vi "Frontpanel.vi"() -> ()   [LabVIEW 2015]
panel:
  in  "stop":bool
  in  "Zeile":u32
  in  "xyz":dbl[](array[numeric])
  in  "Lšschen":bool
  in  "Laden":bool
  in  "Speichern":bool
  in  "Bemerkung":string
  in  "Wellenl.":string
  in  "Favoriten":i32(listbox)
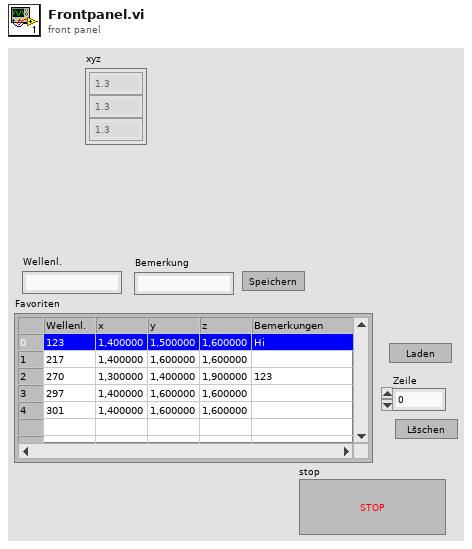
[diagram p1: front panel]
types:
  T1 = enum16{"None", "On Hover", "On Key Focus", "On Hover or Key Focus"}
  T2 = cluster{string[][], "element":string[], string[]}
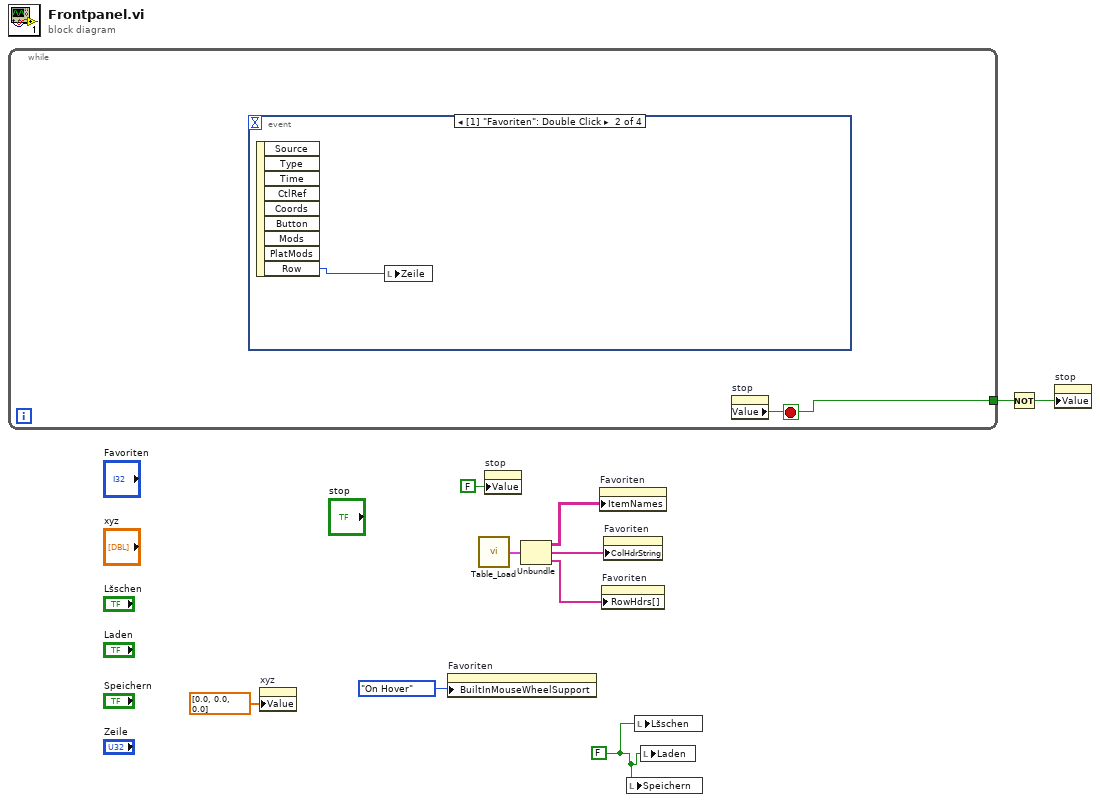
[diagram p0: block diagram]
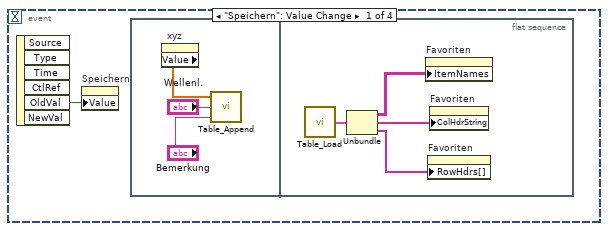
[diagram p2: hidden frame]
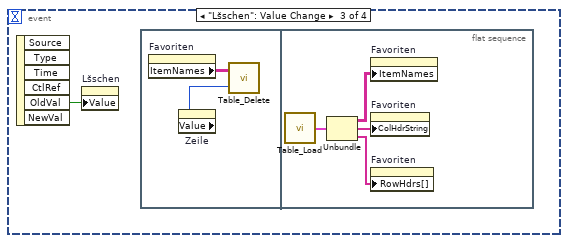
[diagram p3: hidden frame]
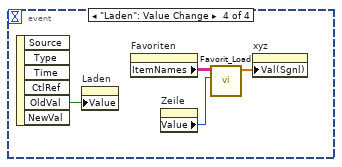
[diagram p4: hidden frame]
diagram:
  w2 = FALSE ("Speichern")
  n1 = while {
    tunnel: [w11] -> w10
    stop <- w11 stop-if-true
    n2 = event shown="[1] \"Favoriten\": Double Click" {
      selector: _ -> [_ _ _ _]
      dyn-events: _ -> [_ _ _ _]
      timeout: _ -> [_ _ _ _]
      event "Speichern": Value Change {
        n3 = event-data() -> ("OldVal"=w12:bool)  [unwired: 1 in, 5 out]
        n4 = property on="Speichern" class="Bool (strict)"("Value"=w12) -> ()  [unwired: 2 in, 2 out]
        n5 = flat-sequence {
          frame #0 {
            n6 = property on="xyz" class="Arr (strict)"() -> ("Value"=w15:dbl[])  [unwired: 2 in, 2 out]
            n7 = call "Table_Append.vi"("Bemerkung"="Bemerkung", "WellenlŠnge"="Wellenl.", "initialized array"=w15) -> ()  [unwired: 1 in]
          }
          frame #1 {
            n8 = call "Table_Load.vi"() -> ("output cluster"=w19:T2)  [unwired: 1 in]
            n9 = Unbundle(w19) -> (w18:string[][], "element"=w16:string[], w17:string[])
            n10 = property on="Favoriten" class="MCListbox (strict)"("ItemNames"=w18) -> ()  [unwired: 2 in, 2 out]
            n11 = property on="Favoriten" class="MCListbox (strict)"("RowHdrs[]"=w17) -> ()  [unwired: 2 in, 2 out]
            n12 = property on="Favoriten" class="MCListbox (strict)"("ColHdrString"=w16) -> ()  [unwired: 2 in, 2 out]
          }
        }
      }
      event "Favoriten": Double Click {
        n13 = event-data() -> ("Row"=w20:i32)  [unwired: 1 in, 8 out]
        n14 = local write "Zeile"(w20) -> ()
      }
      event "Lšschen": Value Change {
        n15 = event-data() -> ("OldVal"=w21:bool)  [unwired: 1 in, 5 out]
        n16 = property on="Lšschen" class="Bool (strict)"("Value"=w21) -> ()  [unwired: 2 in, 2 out]
        n17 = flat-sequence {
          frame #0 {
            n18 = property on="Favoriten" class="MCListbox (strict)"() -> ("ItemNames"=w23:string[][])  [unwired: 2 in, 2 out]
            n19 = property on="Zeile" class="DigNum (strict)"() -> ("Value"=w22:u32)  [unwired: 2 in, 2 out]
            n20 = call "Table_Delete.vi"("Zeile"=w22, "Item Names"=w23) -> ()  [unwired: 1 in]
          }
          frame #1 {
            n21 = call "Table_Load.vi"() -> ("output cluster"=w27:T2)  [unwired: 1 in]
            n22 = Unbundle(w27) -> (w26:string[][], "element"=w24:string[], w25:string[])
            n23 = property on="Favoriten" class="MCListbox (strict)"("ItemNames"=w26) -> ()  [unwired: 2 in, 2 out]
            n24 = property on="Favoriten" class="MCListbox (strict)"("ColHdrString"=w24) -> ()  [unwired: 2 in, 2 out]
            n25 = property on="Favoriten" class="MCListbox (strict)"("RowHdrs[]"=w25) -> ()  [unwired: 2 in, 2 out]
          }
        }
      }
      event "Laden": Value Change {
        n26 = event-data() -> ("OldVal"=w31:bool)  [unwired: 1 in, 5 out]
        n27 = property on="Laden" class="Bool (strict)"("Value"=w31) -> ()  [unwired: 2 in, 2 out]
        n28 = property on="Favoriten" class="MCListbox (strict)"() -> ("ItemNames"=w29:string[][])  [unwired: 2 in, 2 out]
        n29 = property on="Zeile" class="DigNum (strict)"() -> ("Value"=w30:u32)  [unwired: 2 in, 2 out]
        n30 = call "Favorit_Load.vi"("Value"=w30, "ItemNames"=w29) -> ("Array"=w28:dbl[])  [unwired: 9 in]
        n31 = property on="xyz" class="Arr (strict)"("Val(Sgnl)"=w28) -> ()  [unwired: 2 in, 2 out]
      }
    }
    n32 = property on="stop" class="Bool (strict)"() -> ("Value"=w11:bool)  [unwired: 2 in, 2 out]
  }
  n33 = property on="xyz" class="Arr (strict)"("Value"=dbl[] [0.0, 0.0, 0.0] ("Array")) -> ()  [unwired: 2 in, 2 out]
  n34 = property on="Favoriten" class="MCListbox (strict)"("BuiltInMouseWheelSupport"=T1."On Hover" ("Built-In Mouse Wheel Support")) -> ()  [unwired: 2 in, 2 out]
  n35 = call "Table_Load.vi"() -> ("output cluster"=w8:T2)  [unwired: 1 in]
  n36 = property on="stop" class="Bool (strict)"("Value"=FALSE ("stop")) -> ()  [unwired: 2 in, 2 out]
  n37 = Unbundle(w8) -> (w7:string[][], "element"=w5:string[], w6:string[])
  n38 = property on="Favoriten" class="MCListbox (strict)"("ItemNames"=w7) -> ()  [unwired: 2 in, 2 out]
  n39 = property on="Favoriten" class="MCListbox (strict)"("RowHdrs[]"=w6) -> ()  [unwired: 2 in, 2 out]
  n40 = property on="Favoriten" class="MCListbox (strict)"("ColHdrString"=w5) -> ()  [unwired: 2 in, 2 out]
  n41 = local write "Speichern"(w2) -> ()
  n42 = local write "Lšschen"(w2) -> ()
  n43 = local write "Laden"(w2) -> ()
  n44 = Not(x=w10) -> (.not. x?=w9:bool)
  n45 = property on="stop" class="Bool (strict)"("Value"=w9) -> ()  [unwired: 2 in, 2 out]
